vi "MAIN__.vi"() -> ()   [LabVIEW 2015]
uses:
  <vilib>/Utility/error.llb/DialogType.ctl
  <vilib>/NI/Modbus Library/API/Master/Modbus Master.lvclass
panel:
  out "refnum out":refnum<file>
  out "register values":u16[](array[numeric])
  out "Связь блоком управления":bool
  in  "Tab Control":enum32{"УПРАВЛЕНИЕ", "НАСТРОЙКИ"}(tab)
  out "U изм.":dbl=1.0 min=0.0 max=5.0 step=0.01 format="%1.2g"
  out "I изм.":dbl=1.0 min=0.0 max=5.0 step=0.01 format="%1.2g"
  in  "I уст.":dbl=1.0 min=0.0 max=5.0 step=0.01 format="%1.2g"
  in  "U уст.":dbl=1.0 min=0.0 max=40.0 step=1.0 format="%#.0p"
  in  "вых вкл.":bool
  in  "вых выкл.":bool
  in  "полярность":bool
  in  "Порт":u16
  in  "IP":string
  in  "stop":bool
  out "Соед.":refnum<class "Modbus Master.lvclass">
  # "I [A]"
  # "U [В]"
  # "Полярность"
  # "±"
  # "УСТ."
  # "ИЗМ."
  # "УСТ."
  # "ИЗМ."
  # "ВДК-ФИ"
  # "Настройки сети"
types:
  T1 = typedef "DialogType.ctl" = u16
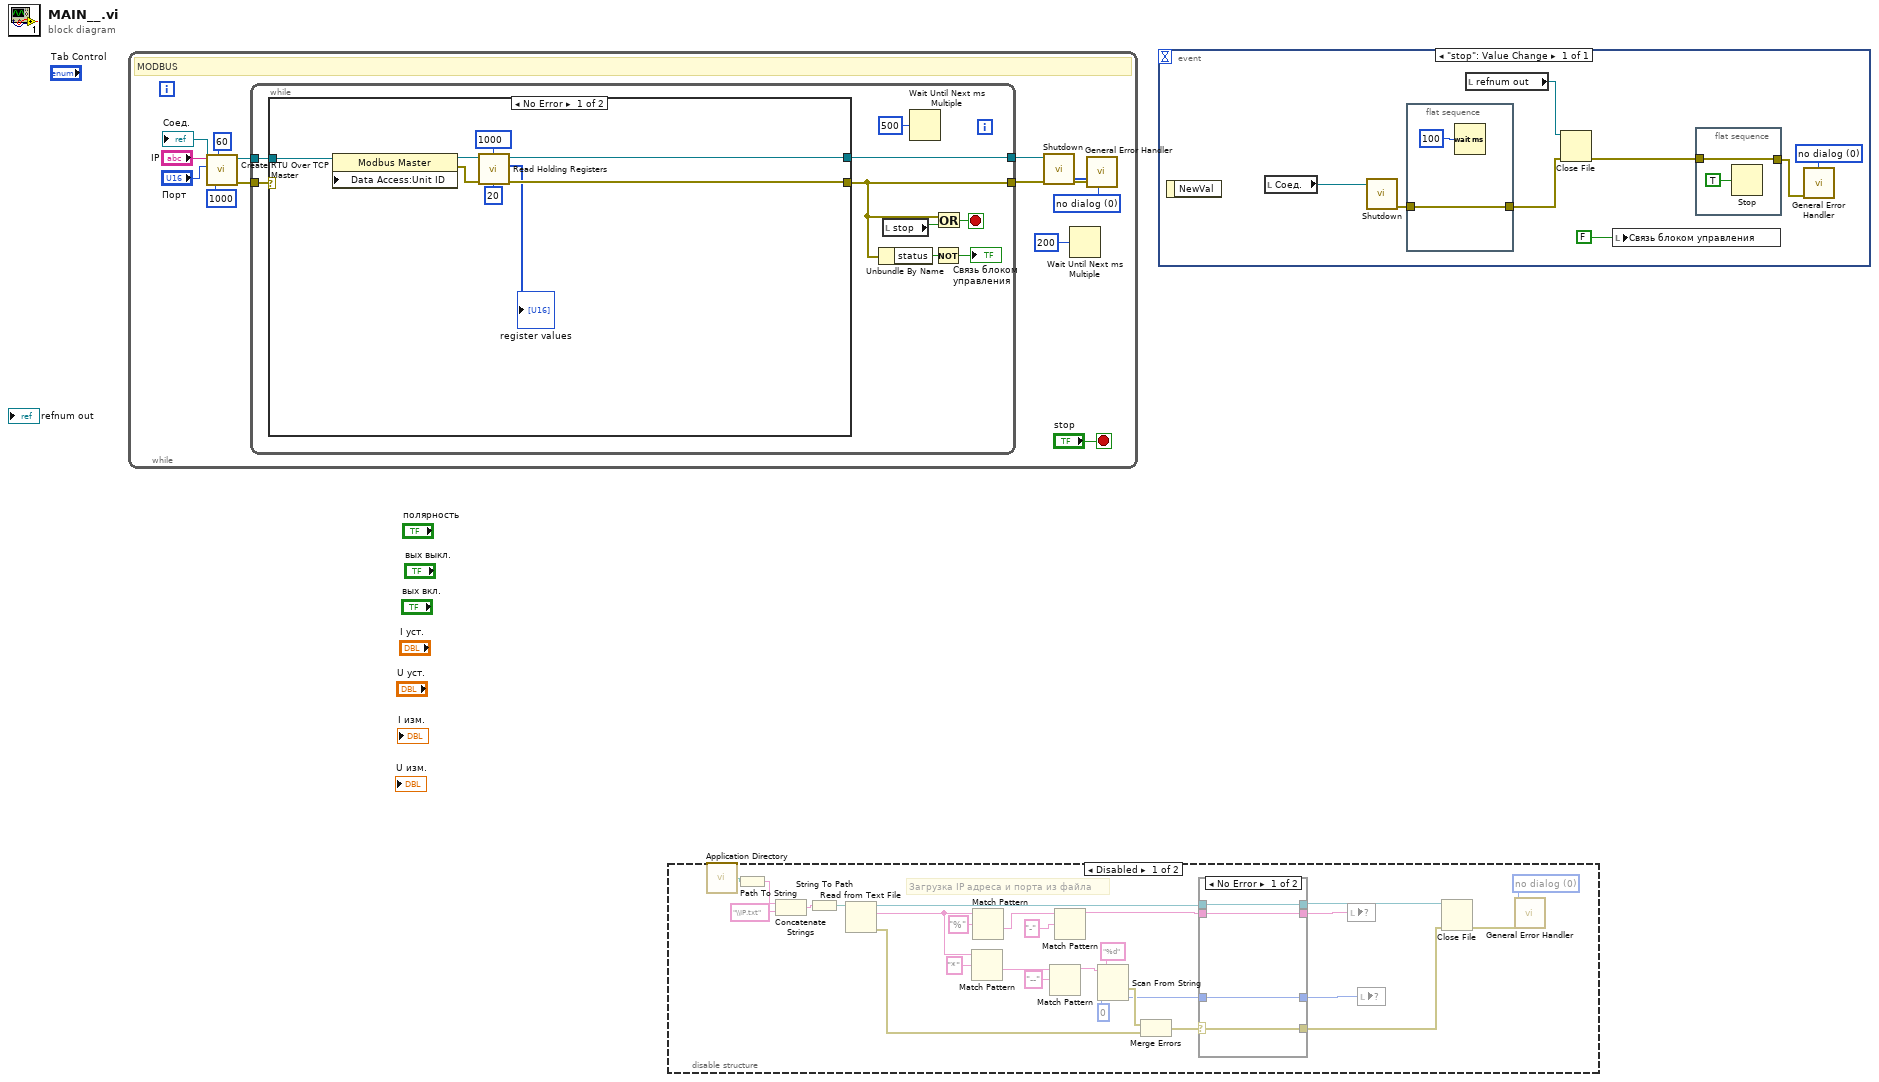
[diagram p0: block diagram]
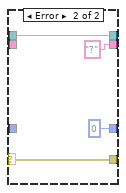
[diagram p2: hidden frame]
diagram:
  n1 = while {
    stop <- "stop" stop-if-true
    w1 = T1 0 items=["no dialog", "OK message", "continue or stop message", "OK message + warnings", "continue/stop + warnings"] ("type of dialog (OK msg:1)")
    # "MODBUS"
    n2 = call "Create RTU Over TCP Master.vi"("unit ID"=u8 60 ("ID"), "connect timeout ms"=1000, "port (502)"="Порт", "address"="IP") -> ("error out"=w5:errorcluster, "TCP master instance"=w6:refnum<class "Modbus Master.lvclass">)  [unwired: 6 in]
    "Соед." <- w6
    n3 = while {
      tunnel: w6 -> [w21]
      tunnel: w5 -> [w20]
      tunnel: [w14] -> w4
      tunnel: [w19] -> w3
      stop <- w17 stop-if-true
      n4 = case shown="No Error" w20 {
        selector: w20 -> [_ w30]
        tunnel: w21 -> [w24 w31]
        tunnel: [w27 w30] -> w14
        tunnel: [w26 w31] -> w19
        frame No Error {
          n5 = property class="Modbus Master" props=["Data Access:Unit ID"](reference=w24) -> (reference out=w23:refnum<class "Modbus Master.lvclass">, error out=w22:errorcluster)  [unwired: 2 in]
          n6 = call-dynamic "Read Holding Registers.vi"("error in"=w22, "number of inputs"=u16 20, "starting address"=u16 1000, "Modbus master in"=w23) -> ("error out"=w27:errorcluster, "register values"=→"register values":u16[], "Modbus master out"=w26:refnum<class "Modbus Master.lvclass">)  [unwired: 5 in]
        }
        frame Error {
        }
      }
      n7 = Unbundle By Name(w14) -> ("status"=w16:bool)
      n8 = local read "stop"() -> (w18:bool)
      n9 = Wait Until Next ms Multiple(millisecond multiple=u32 500) -> ()  [unwired: 1 out]
      n10 = Not(x=w16) -> (.not. x?=→"Связь блоком управления":bool)
      n11 = Or(x=w14, y=w18) -> (x .or. y?=w17:bool)
    }
    n12 = call-dynamic "Shutdown.vi"("error in"=w4, "Modbus master in"=w3) -> ("error out"=w2:errorcluster)  [unwired: 9 in]
    n13 = Wait Until Next ms Multiple(millisecond multiple=u32 200) -> ()  [unwired: 1 out]
    n14 = call <vilib>:"General Error Handler.vi"("type of dialog (OK msg:1)"=w1, "error in (no error)"=w2) -> ()  [unwired: 1 in, 13 out]
  }
  n15 = disable-structure shown="Disabled" {
    frame Disabled {
      w57 = T1 0 items=["no dialog", "OK message", "continue or stop message", "OK message + warnings", "continue/stop + warnings"] ("type of dialog (OK msg:1)")
      # "Загрузка IP адреса и порта из файла"
      n16 = call <vilib>:"Application Directory.vi"() -> ("Application Directory"=w38:path)
      n17 = Path To String(path=w38) -> (string=w37:string)
      n18 = Concatenate Strings(w37, "\\IP.txt" ("prompt (Open existing file)")) -> (w36:string)
      n19 = String To Path(string=w36) -> (path=w34:path)
      n20 = Read from Text File(file (use dialog)=w34) -> (refnum out=w45:refnum<file>, text=w32:string, error out=w58:errorcluster)  [unwired: 3 in, 1 out]
      n21 = Match Pattern(string=w32, regular expression="*") -> (after substring=w53:string)  [unwired: 1 in, 3 out]
      n22 = Match Pattern(string=w32, regular expression="%") -> (after substring=w39:string)  [unwired: 1 in, 3 out]
      n23 = Match Pattern(string=w53, regular expression="--" ("string")) -> (before substring=w54:string)  [unwired: 1 in, 3 out]
      n24 = Match Pattern(string=w39, regular expression="-" ("string")) -> (before substring=w40:string)  [unwired: 1 in, 3 out]
      n25 = Scan From String(format string="%d", input string=w54, default 1=u16 0 ("default value 1")) -> (error out=w55:errorcluster, output 1=w41:u16)  [unwired: 2 in, 2 out]
      n26 = Merge Errors(w55, w58) -> (w42:errorcluster)
      n27 = case shown="No Error" w42 {
        selector: w42 -> [w60 w63]
        tunnel: w40 -> [w62 _]
        tunnel: w41 -> [w61 _]
        tunnel: [w62 "?"] -> w43
        tunnel: [w61 u16 0 ("default value 1")] -> w44
        tunnel: w45 -> [w59 w64]
        tunnel: [w59 w64] -> w46
        tunnel: [w60 w63] -> w47
        frame No Error {
        }
        frame Error {
        }
      }
      n28 = local write item#-1(w43) -> ()
      n29 = local write item#-1(w44) -> ()
      n30 = Close File(refnum=w46, error in=w47) -> (error out=w48:errorcluster)  [unwired: 1 out]
      n31 = call <vilib>:"General Error Handler.vi"("type of dialog (OK msg:1)"=w57, "error in (no error)"=w48) -> ()  [unwired: 1 in, 13 out]
    }
    frame Enabled {
    }
  }
  n32 = event shown="[0] \"stop\": Value Change" {
    selector: _ -> [_]
    dyn-events: _ -> [_]
    timeout: _ -> [_]
    event "stop": Value Change {
      w71 = T1 0 items=["no dialog", "OK message", "continue or stop message", "OK message + warnings", "continue/stop + warnings"] ("type of dialog (OK msg:1)")
      n33 = event-data() -> ()  [unwired: 1 in, 1 out]
      n34 = local read "Соед."() -> (w73:refnum<class "Modbus Master.lvclass">)
      n35 = call-dynamic "Shutdown.vi"("Modbus master in"=w73) -> ("error out"=w72:errorcluster)  [unwired: 10 in]
      n36 = flat-sequence {
        tunnel: w72 -> [w77]
        tunnel: [w77] -> w70
        frame #0 {
          n37 = Wait (ms)(milliseconds to wait=u32 100) -> ()  [unwired: 1 out]
        }
      }
      n38 = local read "refnum out"() -> (w74:refnum<file>)
      n39 = Close File(refnum=w74, error in=w70) -> (error out=w68:errorcluster)  [unwired: 1 out]
      n40 = local write "Связь блоком управления"(FALSE ("Запись в файл")) -> ()
      n41 = flat-sequence {
        tunnel: [w75] -> w67
        tunnel: w68 -> [w75]
        frame #0 {
          n42 = Stop(stop? (T)=TRUE) -> ()
        }
      }
      n43 = call <vilib>:"General Error Handler.vi"("error in (no error)"=w67, "[exception action] (none:0)"=w71) -> ()  [unwired: 2 in, 12 out]
    }
  }
